vi "Core.vi"(11 "Instr in":refnum<class "ePAS.lvclass">) -> ()   [LabVIEW 2014, in "ePAS Library.lvlib" / "ePAS.lvclass"]
uses:
  ePAS.lvclass
  reusable/PAS/Main/PAS.lvclass
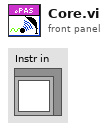
[diagram p1: front panel]
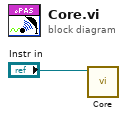
[diagram p0: block diagram]
diagram:
  n1 = call-parent "Core.vi"("Instr in"="Instr in") -> ()  [unwired: 11 in]
